vi "PH_Switch_USB.ProcCases.vi"(0 "i ref in":refnum<vi>, 1 "selector":string, 2 "Data":T1, 3 "call cluster":T2={"Object"="", "Selector"="", "CallType"=enum."synchronous", "Async Object"="", "Async Selector"="", "Data Descriptor"="", "Data"=[], "Error #"=0, "Expire"=0}, 5 "error in (no error)":errorcluster) -> (14 "i ref out":refnum<vi>, 17 "answer cluster":T2={"Object"="", "Selector"="", "CallType"=enum."synchronous", "Async Object"="", "Async Selector"="", "Data Descriptor"="", "Data"=[], "Error #"=0, "Expire"=0}, 19 "error out":errorcluster)   [LabVIEW 2014, in "PH_Switch_USB.lvlib"]
doc: "This method is called by a process from within the default case in the event loop. The methods of a class that are linked to events will be called from THIS method. Add your code here."
uses:
  PH_Switch_USB.lvlib
  CSCore/CSSystem/CoreDefs/CoreDefs.call_type.ctl
  CSCore/BaseProcess/BaseProcess.descriptor string definition.ctl
  CSCore/CSSystem/CoreDefs/CoreDefs.rawDataType.ctl
  CSCore/CSSystem/CoreLib/CoreLib.string 2 byte array.vi
  CSCore/CSSystem/CoreLib/CoreLib.byte array 2 short.vi
  CSCore/CSSystem/CoreLib/CoreLib.int 2 byte array.vi
  CSCore/CSSystem/CoreLib/CoreLib.short 2 byte array.vi
  CSCore/BaseProcess/BaseProcess.lvlib
  CSCore/CSSystem/CoreLib/CoreLib.lvlib
  CSCore/CAEObj/CAEObj.lvlib
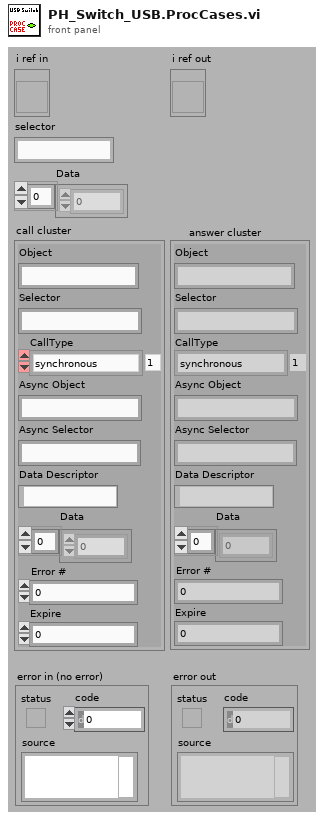
[diagram p1: front panel]
types:
  T1 = typedef "CoreDefs.rawDataType.ctl" = i8[]
  T2 = typedef "CoreDefs.call_type.ctl" = cluster{"Object":string, "Selector":string, "CallType":enum16{"simple", "synchronous", "asynchronous"}, "Async Object":string, "Async Selector":string, "Data Descriptor":T3, "Data":T1, "Error #":i32, "Expire":u32}
  T3 = typedef "BaseProcess.lvlib/BaseProcess.descriptor string definition.ctl" = string
  T4 = typedef "PH_Switch_USB.lvlib/PH_Switch_USB.i attribute.ctl" = cluster{"GUI Refs":cluster{"GUI-Knob":refnum<vi>, "Delete":refnum<vi>}, "Switch":cluster{"GUI Ref":refnum<vi>, "Service name":string, "Array No.":i16, "caption":string, "Status":T5}, "True-Sensor":cluster{"GUI Ref":refnum<vi>, "Service name":string, "Array No.":i16, "caption":string, "Status":T5}, "False-Sensor":cluster{"GUI Ref":refnum<vi>, "Service name":string, "Array No.":i16, "caption":string, "Status":T5}}
  T5 = typedef "PH_StatusHandler.lvlib/PH_StatusHandler.Status.ctl" = i16
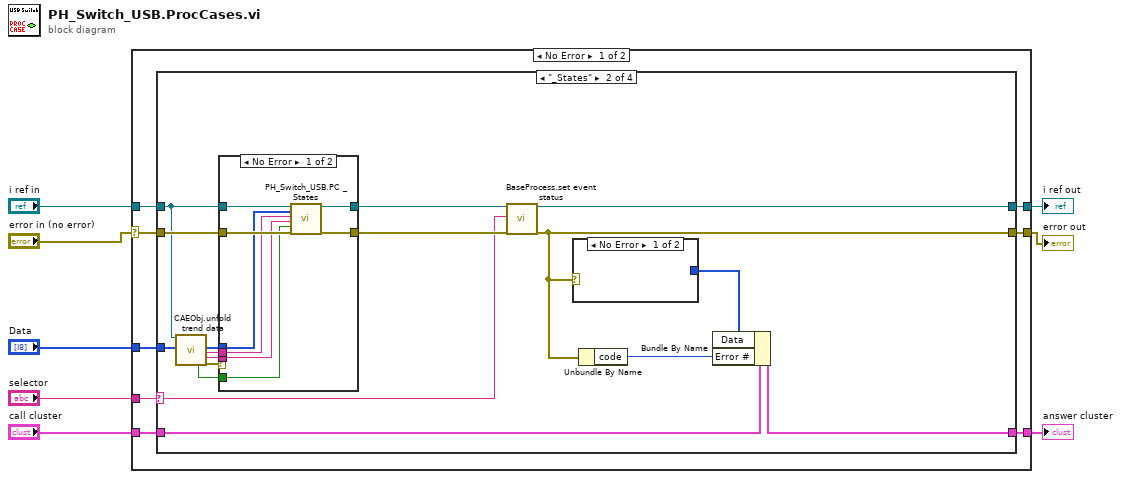
[diagram p0: block diagram]
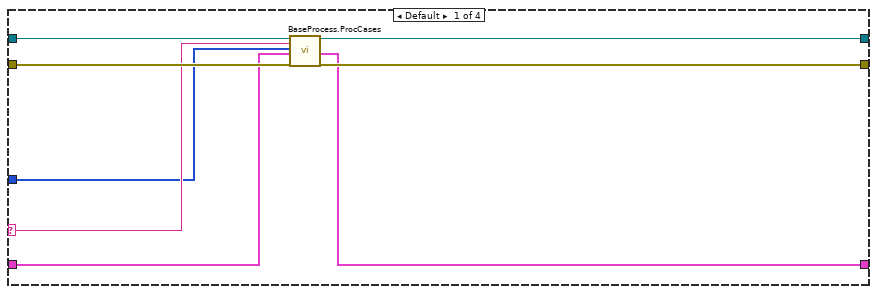
[diagram p2: hidden frame]
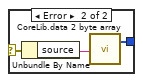
[diagram p4: hidden frame]
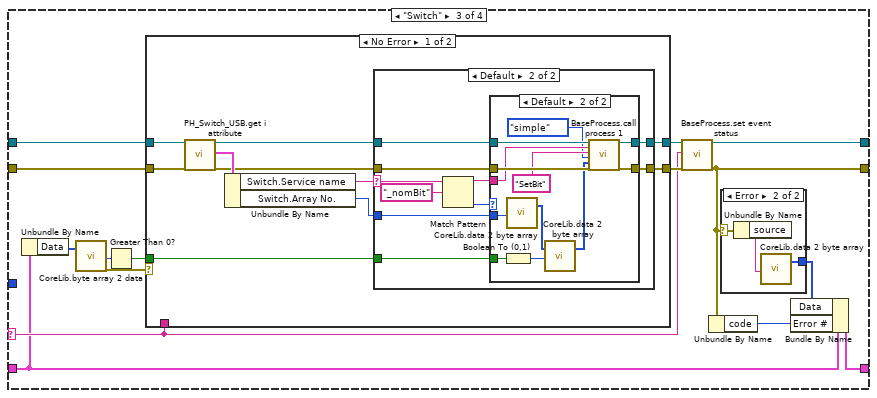
[diagram p5: hidden frame]
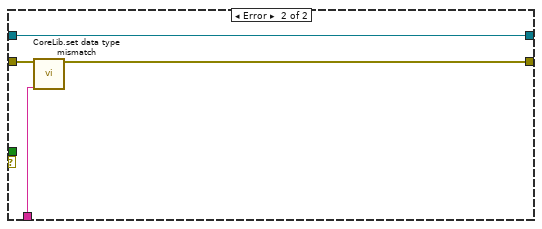
[diagram p9: hidden frame]
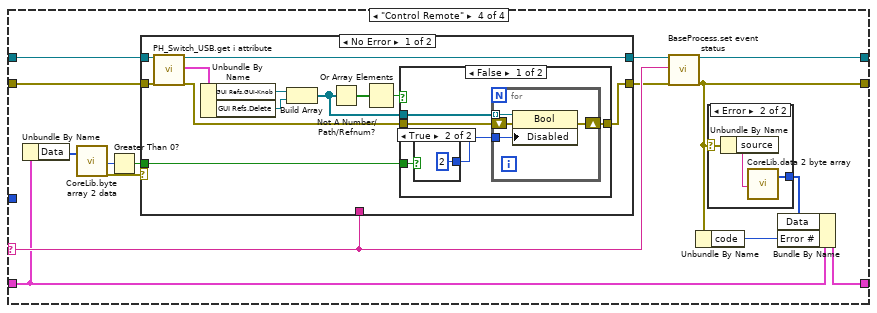
[diagram p10: hidden frame]
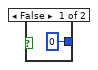
[diagram p12: hidden frame]
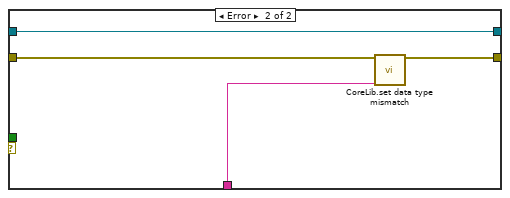
[diagram p14: hidden frame]
diagram:
  n1 = case shown="No Error" "error in (no error)" {
    selector: "error in (no error)" -> [w9 w160]
    tunnel: "selector" -> [w16 _]
    tunnel: [w15 w159] -> w7
    tunnel: "call cluster" -> [w14 w159]
    tunnel: "i ref in" -> [w13 w161]
    tunnel: [w12 w161] -> w4
    tunnel: [w11 w160] -> w3
    tunnel: "Data" -> [w10 _]
    frame No Error {
      n2 = case shown="\"_States\"" w16 {
        selector: w16 -> [w19 w30 w59 w119]
        tunnel: w13 -> [w18 w26 w68 w123]
        tunnel: [w24 w31 w55 w116] -> w12
        tunnel: w14 -> [w20 w29 w58 w113]
        tunnel: [w21 w28 w57 w114] -> w15
        tunnel: w9 -> [w23 w33 w69 w122]
        tunnel: [w22 w32 w56 w115] -> w11
        tunnel: w10 -> [w17 w27 _ _]
        frame Default {
          n3 = call "BaseProcess.ProcCases.vi"("i ref in"=w18, "selector"=w19, "Data"=w17, "call cluster"=w20, "error in (no error)"=w23) -> ("i ref out"=w24:refnum<vi>, "answer cluster"=w21:T2, "error out"=w22:errorcluster)  [unwired: 12 in]
        }
        frame "_States" {
          n4 = call "CAEObj.unfold trend data.vi"("i ref in"=w26, "raw trend data"=w27) -> ("no link"=w37:bool, "data"=w40:i8[], "serviceName"=w25:string, "typeDescriptor"=w38:string, "error out"=w39:errorcluster)  [unwired: 9 in, 4 out]
          n5 = case shown="No Error" w39 {
            tunnel: w33 -> [w46 w50]
            tunnel: [w49 w51] -> w35
            tunnel: [w48 w50] -> w36
            tunnel: w26 -> [w47 w51]
            tunnel: w37 -> [w42 _]
            tunnel: w38 -> [w43 _]
            tunnel: w40 -> [w45 _]
            tunnel: w25 -> [w44 _]
            frame No Error {
              n6 = call "PH_Switch_USB.PC _States.vi"("i ref in"=w47, "data"=w45, "serviceName"=w44, "typeDescriptor"=w43, "no link"=w42, "error IO"=w46) -> ("i ref out"=w49:refnum<vi>, "error out"=w48:errorcluster)  [unwired: 12 in]
            }
            frame Error {
            }
          }
          n7 = call "BaseProcess.set event status.vi"("i ref in"=w35, "EventStatus"=w30, "error in (no error)"=w36) -> ("i ref out"=w31:refnum<vi>, "error out"=w32:errorcluster)  [unwired: 14 in, 1 out]
          n8 = case shown="No Error" w32 {
            selector: w32 -> [_ w54]
            tunnel: [_ w52] -> w41
            frame No Error {
            }
            frame Error {
              n9 = Unbundle By Name(w54) -> ("source"=w53:string)
              n10 = call-poly "CoreLib.data 2 byte array.vi"("string"=w53) -> ("byteArray out"=w52:T1)  [unwired: 18 in]
            }
          }
          n11 = Unbundle By Name(w32) -> ("code"=w34:i32)
          n12 = Bundle By Name(cluster=w29, "Data"=w41, "Error #"=w34) -> (w28:T2)
        }
        frame "Switch" {
          n13 = Unbundle By Name(w58) -> ("Data"=w67:T1)
          n14 = call-poly "CoreLib.byte array 2 data.vi"("byteArray"=w67) -> ("i16"=w66:i16, "error out"=w65:errorcluster)  [unwired: 16 in, 1 out]
          n15 = Greater Than 0?(x=w66) -> (x > 0?=w64:bool)
          n16 = case shown="No Error" w65 {
            tunnel: [w77 w112] -> w61
            tunnel: [w76 w109] -> w60
            tunnel: w68 -> [w82 w112]
            tunnel: w69 -> [w81 w111]
            tunnel: w59 -> [_ w110]
            tunnel: w64 -> [w74 _]
            frame No Error {
              n17 = call "PH_Switch_USB.get i attribute.vi"("i ref in"=w82, "error in (no error)"=w81) -> ("i ref out"=w78:refnum<vi>, "i attribute"=w80:T4, "error out"=w79:errorcluster)  [unwired: 15 in]
              n18 = Unbundle By Name(w80) -> ("Switch.Service name"=w73:string, "Switch.Array No."=w75:i16)
              n19 = case shown="Default" w73 {
                selector: w73 -> [_ w85]
                tunnel: w79 -> [w83 w94]
                tunnel: w78 -> [w84 w93]
                tunnel: [w84 w92] -> w77
                tunnel: [w83 w91] -> w76
                tunnel: w75 -> [_ w87]
                tunnel: w74 -> [_ w86]
                frame "", "N/A" {
                }
                frame Default {
                  n20 = Match Pattern(string=w85, regular expression="_nomBit") -> (before substring=w88:string, offset past match=w89:i32)  [unwired: 1 in, 2 out]
                  n21 = case shown="Default" w89 {
                    tunnel: w94 -> [w95 w108]
                    tunnel: w93 -> [w96 w107]
                    tunnel: [w96 w106] -> w92
                    tunnel: [w95 w105] -> w91
                    tunnel: w88 -> [_ w104]
                    tunnel: w87 -> [_ w101]
                    tunnel: w86 -> [_ w100]
                    frame -1 {
                    }
                    frame Default {
                      n22 = Boolean To (0,1)(Boolean=w100) -> (0, 1=w102:i16)
                      n23 = call-poly "CoreLib.data 2 byte array.vi"("i32"=w101) -> ("byteArray out"=w99:T1)  [unwired: 18 in]
                      n24 = call-poly "CoreLib.data 2 byte array.vi"("byteArray"=w99, "i16"=w102) -> ("byteArray out"=w98:T1)  [unwired: 17 in]
                      n25 = call "BaseProcess.call process 1.vi"("i ref in"=w107, "Object"=w104, "Selector"="SetBit", "CallType"=enum16{"simple", "synchronous", "asynchronous"}."simple", "Data"=w98, "error in (no error)"=w108) -> ("i ref out"=w106:refnum<vi>, "error out"=w105:errorcluster)  [unwired: 11 in, 1 out]
                    }
                  }
                }
              }
            }
            frame Error {
              n26 = call "CoreLib.set data type mismatch.vi"("error in (no error)"=w111, "error source"=w110) -> ("error out"=w109:errorcluster)  [unwired: 17 in]
            }
          }
          n27 = call "BaseProcess.set event status.vi"("i ref in"=w61, "EventStatus"=w59, "error in (no error)"=w60) -> ("i ref out"=w55:refnum<vi>, "error out"=w56:errorcluster)  [unwired: 14 in, 1 out]
          n28 = Unbundle By Name(w56) -> ("code"=w63:i32)
          n29 = case shown="Error" w56 {
            selector: w56 -> [_ w72]
            tunnel: [_ w70] -> w62
            frame No Error {
            }
            frame Error {
              n30 = Unbundle By Name(w72) -> ("source"=w71:string)
              n31 = call-poly "CoreLib.data 2 byte array.vi"("string"=w71) -> ("byteArray out"=w70:T1)  [unwired: 18 in]
            }
          }
          n32 = Bundle By Name(cluster=w58, "Data"=w62, "Error #"=w63) -> (w57:T2)
        }
        frame "Control Remote" {
          n33 = Unbundle By Name(w113) -> ("Data"=w124:T1)
          n34 = call-poly "CoreLib.byte array 2 data.vi"("byteArray"=w124) -> ("i16"=w125:i16, "error out"=w127:errorcluster)  [unwired: 16 in, 1 out]
          n35 = Greater Than 0?(x=w125) -> (x > 0?=w126:bool)
          n36 = case shown="No Error" w127 {
            tunnel: [w138 w158] -> w118
            tunnel: w123 -> [w142 w158]
            tunnel: w122 -> [w141 w157]
            tunnel: [w137 w156] -> w117
            tunnel: w119 -> [_ w155]
            tunnel: w126 -> [w136 _]
            frame No Error {
              n37 = call "PH_Switch_USB.get i attribute.vi"("i ref in"=w142, "error in (no error)"=w141) -> ("i ref out"=w138:refnum<vi>, "i attribute"=w140:T4, "error out"=w139:errorcluster)  [unwired: 15 in]
              n38 = Unbundle By Name(w140) -> ("GUI Refs.GUI-Knob"=w135:refnum<vi>, "GUI Refs.Delete"=w134:refnum<vi>)
              n39 = Build Array(w135, w134) -> (w133:refnum<vi>[])
              n40 = Not A Number/Path/Refnum?(number/path/refnum=w133) -> (NaN/Path/Refnum?=w132:bool[])
              n41 = Or Array Elements(Boolean array=w132) -> (logical OR=w131:bool)
              n42 = case shown="False" w131 {
                tunnel: w133 -> [w147 _]
                tunnel: w139 -> [w146 w154]
                tunnel: [w145 w154] -> w137
                tunnel: w136 -> [w144 _]
                frame False {
                  n43 = case shown="True" w144 {
                    tunnel: [0 2] -> w143
                    frame False {
                    }
                    frame True {
                    }
                  }
                  n44 = for {
                    tunnel: w147 -> [w151] mode=indexing
                    tunnel: w143 -> [w148]
                    shift-right: [w149] -> w145
                    shift-left: w146 -> [w150]
                    n45 = property class="Bool"(reference=w151, error in=w150, "Disabled"=w148) -> (error out=w149:errorcluster)  [unwired: 1 out]
                  }
                }
                frame True {
                }
              }
            }
            frame Error {
              n46 = call "CoreLib.set data type mismatch.vi"("error in (no error)"=w157, "error source"=w155) -> ("error out"=w156:errorcluster)  [unwired: 17 in]
            }
          }
          n47 = call "BaseProcess.set event status.vi"("i ref in"=w118, "EventStatus"=w119, "error in (no error)"=w117) -> ("i ref out"=w116:refnum<vi>, "error out"=w115:errorcluster)  [unwired: 14 in, 1 out]
          n48 = Unbundle By Name(w115) -> ("code"=w121:i32)
          n49 = case shown="Error" w115 {
            selector: w115 -> [_ w130]
            tunnel: [_ w128] -> w120
            frame No Error {
            }
            frame Error {
              n50 = Unbundle By Name(w130) -> ("source"=w129:string)
              n51 = call-poly "CoreLib.data 2 byte array.vi"("string"=w129) -> ("byteArray out"=w128:T1)  [unwired: 18 in]
            }
          }
          n52 = Bundle By Name(cluster=w113, "Data"=w120, "Error #"=w121) -> (w114:T2)
        }
      }
    }
    frame Error {
    }
  }
  "answer cluster" <- w7
  "i ref out" <- w4
  "error out" <- w3
